vi "Handle Value Change - Add to Project.vi"(8 "Error In":errorcluster, 10 "New Value":bool, 11 "Module Data In":T1) -> (0 "Error Out":errorcluster)   [LabVIEW 2022 SP3]
doc: "This VI handles the Value Change event on the \"Add To Project?\" checkbox.\n\nAcronyms\nATP = \"Add To Project?\" checkbox\nATO = \"Add To Owner?\" checkbox\nATVF = \"Add To Virtual Folder?\" checkbox"
uses:
  Module Data.ctl
  GUI Object Refs (cluster).ctl
  Initial State (enum).ctl
  Input Conditions (cluster).ctl
  DFS Output (cluster).ctl
panel:
  # "Development\nControls or indicators that are useful for development or testing, but which are not outputs of the VI."
  # "Input\nInputs to the VI"
  # "Output\nOutputs of the VI"
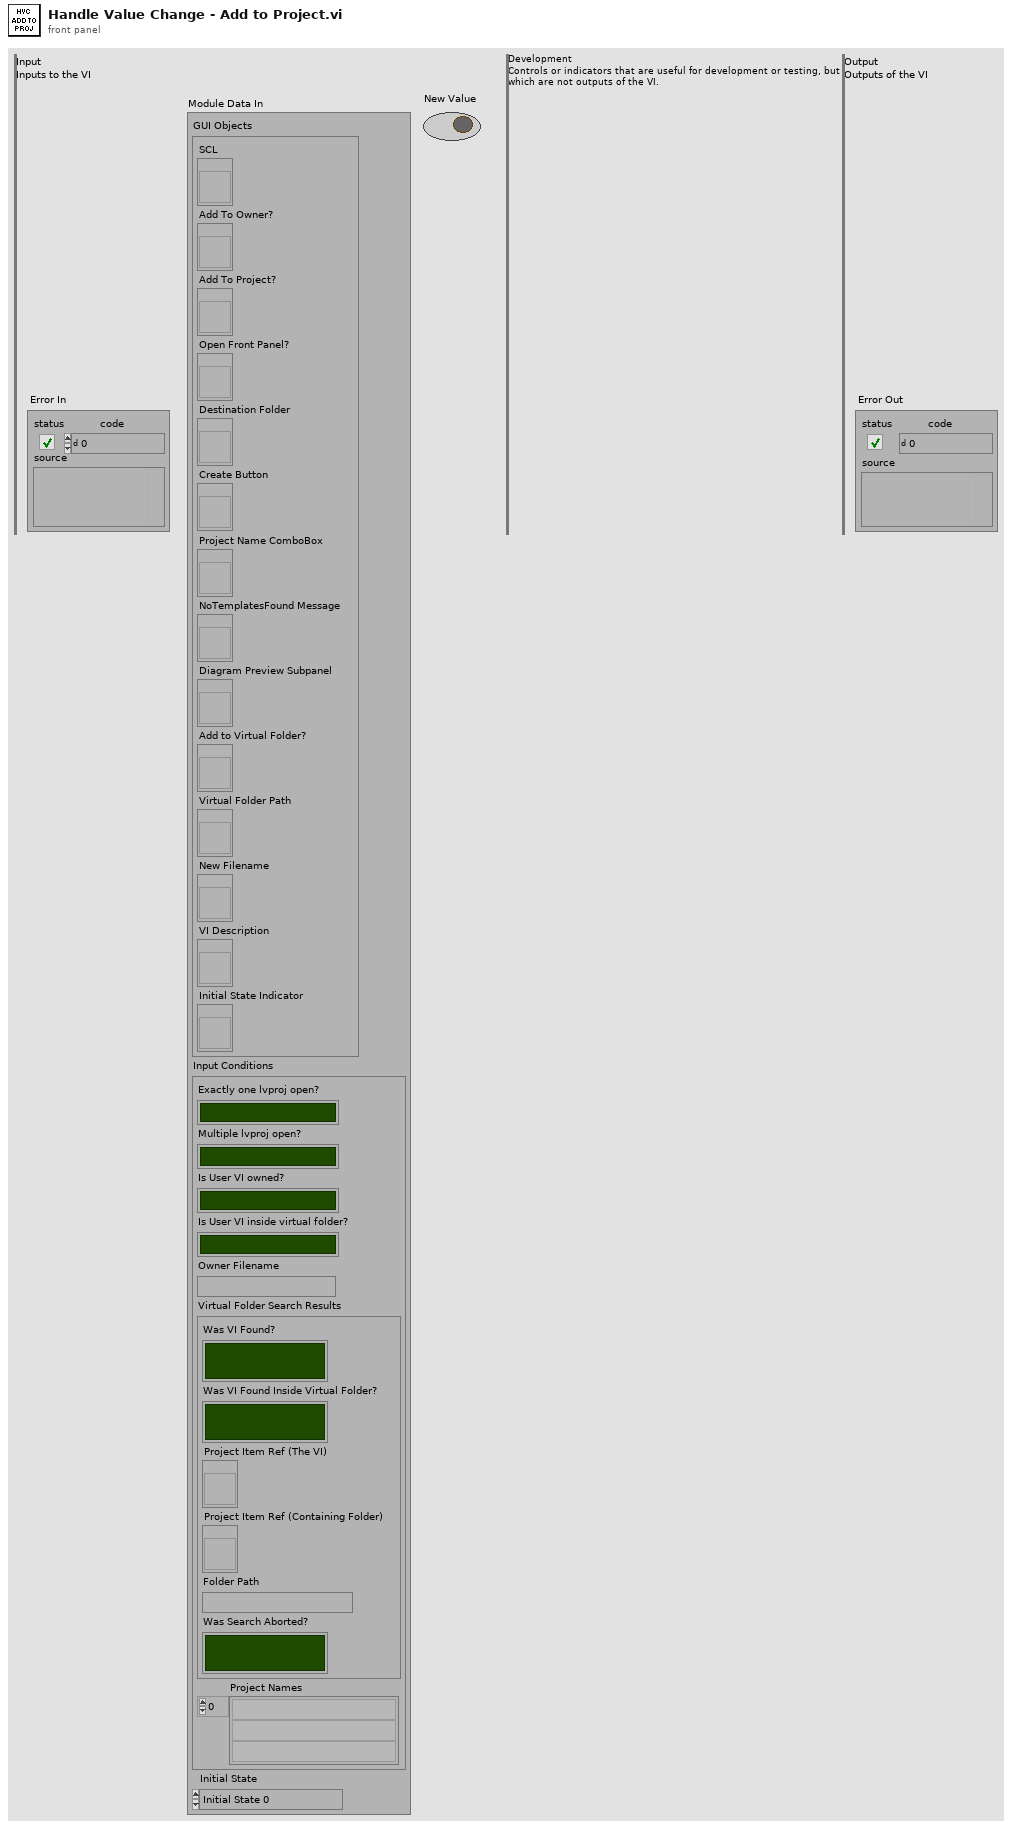
[diagram p1: front panel]
types:
  T1 = typedef "Module Data.ctl" = cluster{"GUI Objects":T2, "Input Conditions":T3, "Initial State":T5}
  T2 = typedef "GUI Object Refs (cluster).ctl" = cluster{"SCL":refnum<vi>, "Add To Owner?":refnum<vi>, "Add To Project?":refnum<vi>, "Open Front Panel?":refnum<vi>, "Destination Folder":refnum<vi>, "Create Button":refnum<vi>, "Project Name ComboBox":refnum<vi>, "NoTemplatesFound Message":refnum<vi>, "Diagram Preview Subpanel":refnum<vi>, "Add to Virtual Folder?":refnum<vi>, "Virtual Folder Path":refnum<vi>, "New Filename":refnum<vi>, "VI Description":refnum<vi>, "Initial State Indicator":refnum<vi>}
  T3 = typedef "Input Conditions (cluster).ctl" = cluster{"Exactly one lvproj open?":bool, "Multiple lvproj open?":bool, "Is User VI owned?":bool, "Is User VI inside virtual folder?":bool, "Owner Filename":string, "Virtual Folder Search Results":T4, "Project Names":string[]}
  T4 = typedef "DFS Output (cluster).ctl" = cluster{"Was VI Found?":bool, "Was VI Found Inside Virtual Folder?":bool, "Project Item Ref (The VI)":refnum<vi>, "Project Item Ref (Containing Folder)":refnum<vi>, "Folder Path":string, "Was Search Aborted?":bool}
  T5 = typedef "Initial State (enum).ctl" = enum16{"Initial State 0", "Initial State 1", "Initial State 2", "Initial State 3", "Initial State 4", "Initial State 5", "Initial State 6", "Initial State 7", "Initial State 8", "Initial State 9", "Initial State 10", "Initial State 11", "Initial State 12", "Initial State 13", "Initial State 14", "Initial State 15"}
  T6 = enum8{"Enabled", "Disabled", "Disabled and Grayed Out"}
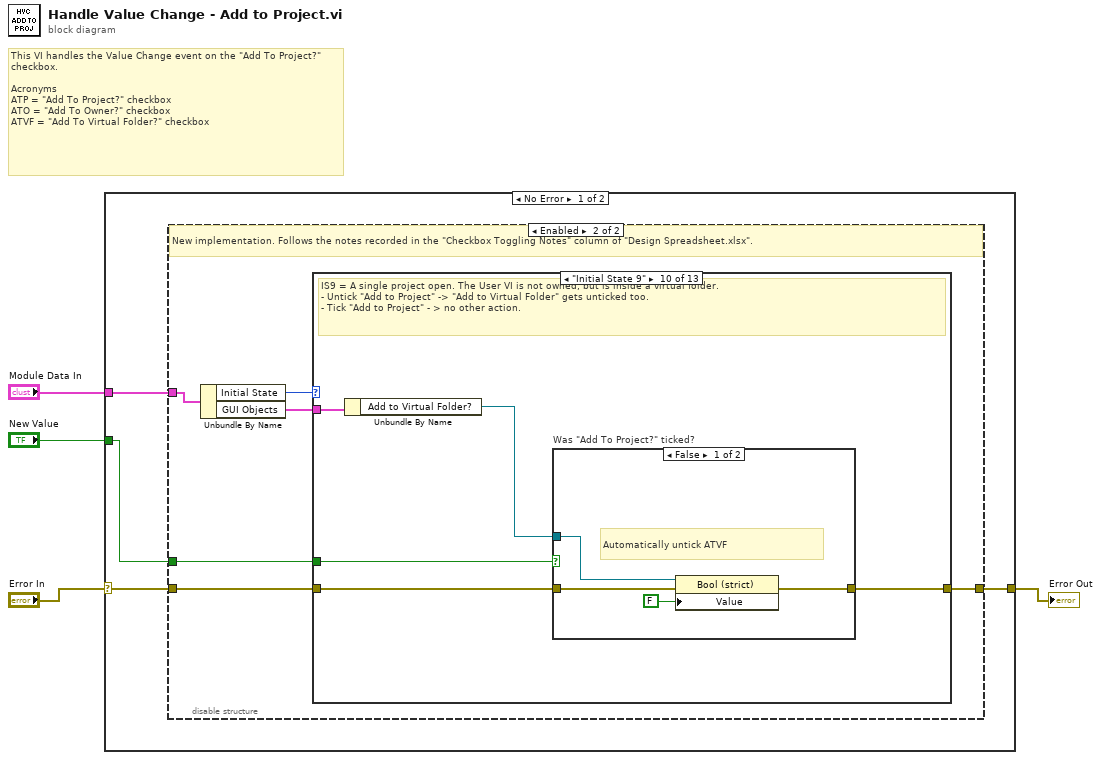
[diagram p0: block diagram]
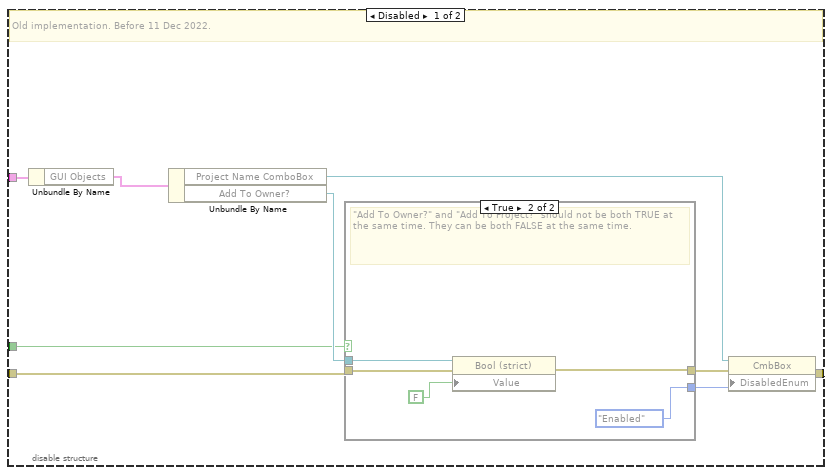
[diagram p2: hidden frame]
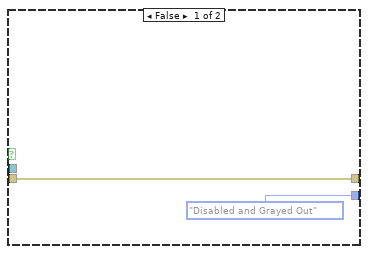
[diagram p3: hidden frame]
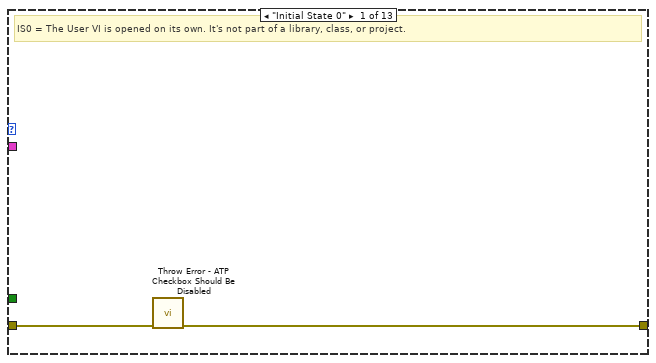
[diagram p4: hidden frame]
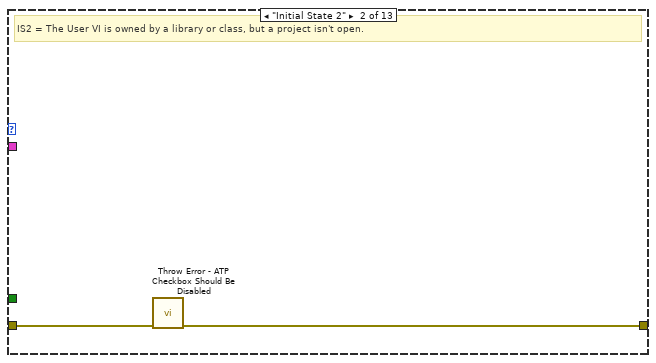
[diagram p5: hidden frame]
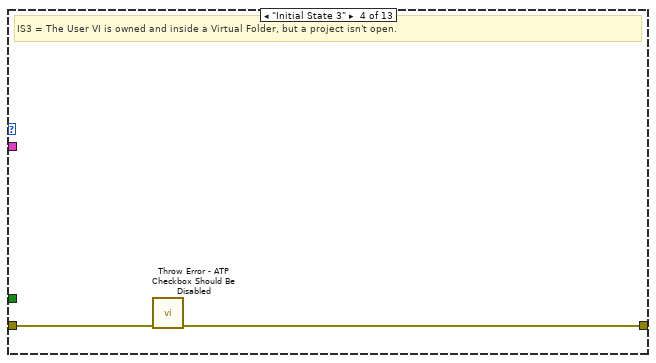
[diagram p7: hidden frame]
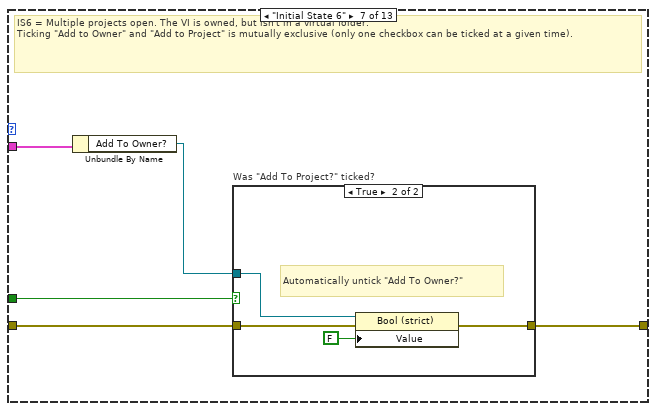
[diagram p10: hidden frame]
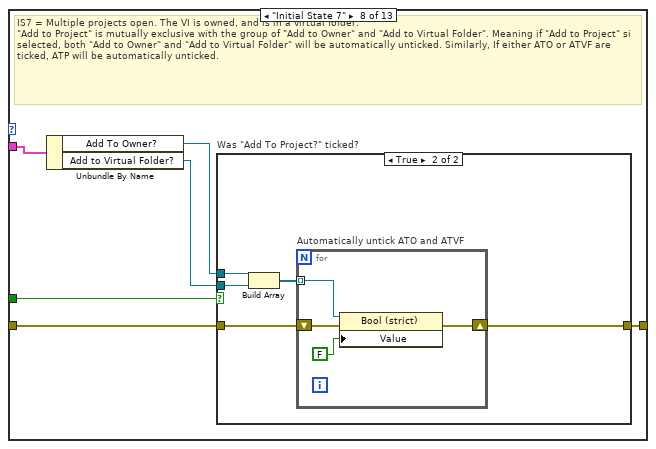
[diagram p12: hidden frame]
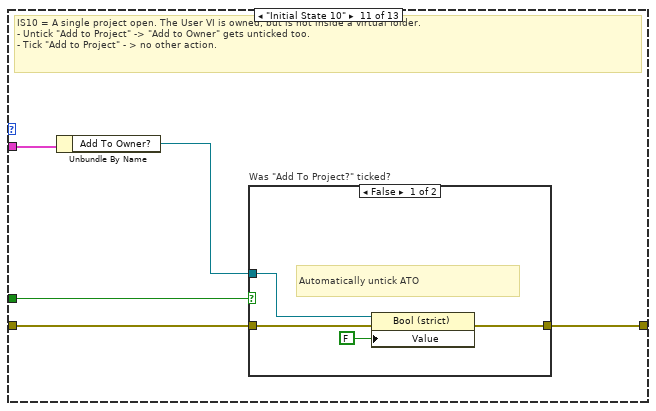
[diagram p16: hidden frame]
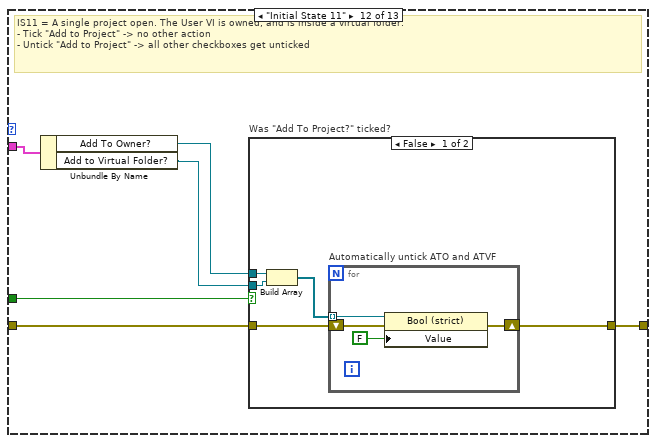
[diagram p18: hidden frame]
diagram:
  # "This VI handles the Value Change event on the \"Add To Project?\" checkbox.\n\nAcronyms\nATP = \"Add To Project?\" checkbox\nATO = \"Add To Owner?\" checkbox\nATVF = \"Add To Virtual Folder?\" checkbox"
  n1 = case shown="No Error" "Error In" {
    selector: "Error In" -> [w8 w104]
    tunnel: [w7 w104] -> w3
    tunnel: "Module Data In" -> [w6 _]
    tunnel: "New Value" -> [w5 _]
    frame No Error {
      n2 = disable-structure shown="Enabled" {
        disable-tunnel: w8 -> [w12 w30]
        disable-tunnel: [w11 w28] -> w7
        disable-tunnel: w6 -> [w10 w29]
        disable-tunnel: w5 -> [w9 w26]
        frame Disabled {
          # "Old implementation. Before 11 Dec 2022."
          n3 = Unbundle By Name(w10) -> ("GUI Objects"=w14:T2)
          n4 = Unbundle By Name(w14) -> ("Project Name ComboBox"=w16:refnum<vi>, "Add To Owner?"=w13:refnum<vi>)
          n5 = case shown="True" w9 {
            tunnel: w12 -> [w19 w23]
            tunnel: [w19 w22] -> w17
            tunnel: [T6."Disabled and Grayed Out" ("Disabled") T6."Enabled" ("Disabled")] -> w15
            tunnel: w13 -> [_ w21]
            frame False {
            }
            frame True {
              # "\"Add To Owner?\" and \"Add To Project?\" should not be both TRUE at the same time. They can be both FALSE at the same time."
              n6 = property class="Bool (strict)"(reference=w21, error in=w23, "Value"=FALSE ("Add To Project?")) -> (error out=w22:errorcluster)  [unwired: 1 out]
            }
          }
          n7 = property class="CmbBox"(reference=w16, error in=w17, "DisabledEnum"=w15) -> (error out=w11:errorcluster)  [unwired: 1 out]
        }
        frame Enabled {
          # "New implementation. Follows the notes recorded in the \"Checkbox Toggling Notes\" column of \"Design Spreadsheet.xlsx\"."
          n8 = Unbundle By Name(w29) -> ("Initial State"=w27:T5, "GUI Objects"=w25:T2)
          n9 = case shown="\"Initial State 9\"" w27 {
            tunnel: w30 -> [w32 w34 w35 w37 w38 w39 w44 w54 w66 w70 w80 w91 w103]
            tunnel: [w31 w33 w35 w36 w38 w39 w43 w53 w66 w67 w77 w88 w103] -> w28
            tunnel: w26 -> [_ _ _ _ _ _ w42 w52 _ w69 w79 w90 _]
            tunnel: w25 -> [_ _ _ _ _ _ w41 w51 _ w68 w78 w89 _]
            frame "Initial State 0" {
              # "IS0 = The User VI is opened on its own. It's not part of a library, class, or project."
              n10 = call "Throw Error - ATP Checkbox Should Be Disabled.vi"("error in"=w32) -> ("error out"=w31:errorcluster)  [unwired: 10 in]
            }
            frame "Initial State 2" {
              # "IS2 = The User VI is owned by a library or class, but a project isn't open."
              n11 = call "Throw Error - ATP Checkbox Should Be Disabled.vi"("error in"=w34) -> ("error out"=w33:errorcluster)  [unwired: 10 in]
            }
            frame "Initial State 1" {
              # "Impossible Initial State. Expected to never occur."
            }
            frame "Initial State 3" {
              # "IS3 = The User VI is owned and inside a Virtual Folder, but a project isn't open."
              n12 = call "Throw Error - ATP Checkbox Should Be Disabled.vi"("error in"=w37) -> ("error out"=w36:errorcluster)  [unwired: 10 in]
            }
            frame "Initial State 4" {
              # "All other checkboxes are disabled, so can't be ticked or unticked. Do nothing."
              # "IS4 = There are multiple projects open. The User VI is likely inside one of the open projects, but we don't know which one. The User VI isn't owned, and isn't in a virtual folder."
            }
            frame "Initial State 5" {
              # "Impossible Initial State. Expected to never occur."
            }
            frame "Initial State 6" {
              # "IS6 = Multiple projects open. The VI is owned, but isn't in a virtual folder.\nTicking \"Add to Owner\" and \"Add to Project\" is mutually exclusive (only one checkbox can be ticked at a given time)."
              n13 = Unbundle By Name(w41) -> ("Add To Owner?"=w40:refnum<vi>)
              n14 = case "Was \"Add To Project?\" ticked?" shown="True" w42 {
                tunnel: w44 -> [w45 w49]
                tunnel: [w45 w48] -> w43
                tunnel: w40 -> [_ w47]
                frame False {
                  # "Do nothing. Don't automatically tick \"Add To Owner?\"."
                }
                frame True {
                  # "Automatically untick \"Add To Owner?\""
                  n15 = property class="Bool (strict)"(reference=w47, error in=w49, "Value"=FALSE) -> (error out=w48:errorcluster)  [unwired: 1 out]
                }
              }
            }
            frame "Initial State 7" {
              # "IS7 = Multiple projects open. The VI is owned, and is in a virtual folder.\n\"Add to Project\" is mutually exclusive with the group of \"Add to Owner\" and \"Add to Virtual Folder\". Meaning if \"Add to Project\" si selected, both \"Add to Owner\" and \"Add to Virtual Folder\" will be automatically unticked. Similarly, If either ATO or ATVF are ticked, ATP will be automatically unticked."
              n16 = Unbundle By Name(w51) -> ("Add To Owner?"=w55:refnum<vi>, "Add to Virtual Folder?"=w50:refnum<vi>)
              n17 = case "Was \"Add To Project?\" ticked?" shown="True" w52 {
                tunnel: [w56 w60] -> w53
                tunnel: w55 -> [_ w59]
                tunnel: w54 -> [w56 w61]
                tunnel: w50 -> [_ w58]
                frame False {
                  # "Do nothing."
                }
                frame True {
                  n18 = Build Array(w59, w58) -> (w57:refnum<vi>[])
                  n19 = for "Automatically untick ATO and ATVF" {
                    shift-right: [w64] -> w60
                    shift-left: w61 -> [w65]
                    tunnel: w57 -> [w62] mode=indexing
                    n20 = property class="Bool (strict)"(reference=w62, error in=w65, "Value"=FALSE) -> (error out=w64:errorcluster)  [unwired: 1 out]
                  }
                }
              }
            }
            frame "Initial State 8" {
              # "All other checkboxes are disabled. Do nothing."
              # "IS8 = A single project open. The User VI is not owned, and is not inside a virtual folder."
            }
            frame "Initial State 9" {
              # "IS9 = A single project open. The User VI is not owned, but is inside a virtual folder.\n- Untick \"Add to Project\" -> \"Add to Virtual Folder\" gets unticked too.\n- Tick \"Add to Project\" - > no other action."
              n21 = Unbundle By Name(w68) -> ("Add to Virtual Folder?"=w71:refnum<vi>)
              n22 = case "Was \"Add To Project?\" ticked?" shown="False" w69 {
                tunnel: w70 -> [w75 w76]
                tunnel: [w74 w76] -> w67
                tunnel: w71 -> [w73 _]
                frame False {
                  # "Automatically untick ATVF"
                  n23 = property class="Bool (strict)"(reference=w73, error in=w75, "Value"=FALSE) -> (error out=w74:errorcluster)  [unwired: 1 out]
                }
                frame True {
                  # "Do nothing."
                }
              }
            }
            frame "Initial State 10" {
              # "IS10 = A single project open. The User VI is owned, but is not inside a virtual folder.\n- Untick \"Add to Project\" -> \"Add to Owner\" gets unticked too.\n- Tick \"Add to Project\" - > no other action."
              n24 = Unbundle By Name(w78) -> ("Add To Owner?"=w81:refnum<vi>)
              n25 = case "Was \"Add To Project?\" ticked?" shown="False" w79 {
                tunnel: w80 -> [w85 w86]
                tunnel: [w84 w86] -> w77
                tunnel: w81 -> [w83 _]
                frame False {
                  # "Automatically untick ATO"
                  n26 = property class="Bool (strict)"(reference=w83, error in=w85, "Value"=FALSE) -> (error out=w84:errorcluster)  [unwired: 1 out]
                }
                frame True {
                  # "Do nothing."
                }
              }
            }
            frame "Initial State 11" {
              # "IS11 = A single project open. The User VI is owned, and is inside a virtual folder.\n- Tick \"Add to Project\" -> no other action\n- Untick \"Add to Project\" -> all other checkboxes get unticked"
              n27 = Unbundle By Name(w89) -> ("Add To Owner?"=w92:refnum<vi>, "Add to Virtual Folder?"=w87:refnum<vi>)
              n28 = case "Was \"Add To Project?\" ticked?" shown="False" w90 {
                tunnel: w91 -> [w97 w102]
                tunnel: [w96 w102] -> w88
                tunnel: w92 -> [w95 _]
                tunnel: w87 -> [w93 _]
                frame False {
                  n29 = Build Array(w95, w93) -> (w94:refnum<vi>[])
                  n30 = for "Automatically untick ATO and ATVF" {
                    tunnel: w94 -> [w99] mode=indexing
                    shift-right: [w100] -> w96
                    shift-left: w97 -> [w101]
                    n31 = property class="Bool (strict)"(reference=w99, error in=w101, "Value"=FALSE) -> (error out=w100:errorcluster)  [unwired: 1 out]
                  }
                }
                frame True {
                  # "Do nothing."
                }
              }
            }
            frame "Initial State 12".."Initial State 15" {
              # "Impossible Initial State. Expected to never occur."
            }
          }
        }
      }
    }
    frame Error {
    }
  }
  "Error Out" <- w3
